vi "dfd_Maxflat API Conversion.vi"(9 "denominator order in":i32, 10 "numerator order in":i32, 11 "filter type":enum16{"IIR", "FIR", "Symmetric FIR"}(ring)) -> (1 "denominator order out":i32, 2 "numerator order out":i32, 3 "symmetric FIR ? (T)":bool)   [LabVIEW 2017, in "NI_DigFilter_Design.lvlib"]
uses:
  <vilib>/addons/Digital Filter Design/NI_DigFilter_Design.lvlib
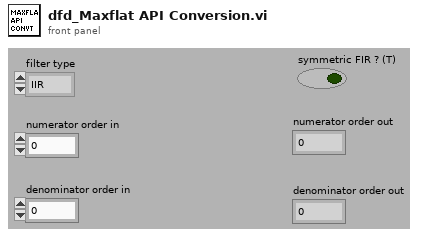
[diagram p1: front panel]
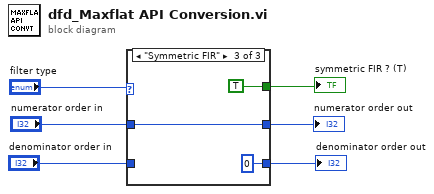
[diagram p0: block diagram]
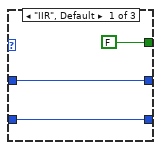
[diagram p2: hidden frame]
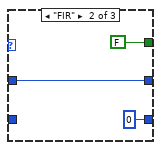
[diagram p3: hidden frame]
diagram:
  n1 = case shown="\"Symmetric FIR\"" "filter type" {
    tunnel: [w9 w11 w14] -> w3
    tunnel: "numerator order in" -> [w9 w11 w14]
    tunnel: "denominator order in" -> [w8 _ _]
    tunnel: [w8 0 ("denominator order") 0 ("denominator order")] -> w5
    tunnel: [FALSE ("symmetric FIR ? (T)") FALSE ("symmetric FIR ? (T)") TRUE ("symmetric FIR ? (T)")] -> w6
    frame "IIR", Default {
    }
    frame "FIR" {
    }
    frame "Symmetric FIR" {
    }
  }
  "symmetric FIR ? (T)" <- w6
  "denominator order out" <- w5
  "numerator order out" <- w3
